vi "CRC16string气密机一.vi"(1 "数组":u16[](array[numeric]) format="%x") -> (0 "要发送的数据":string)   [LabVIEW 2014]
panel:
  out "交换后的校验和":u16 format="%x"
  out "校验和":i32 format="%x"
  out "数组个数":dbl
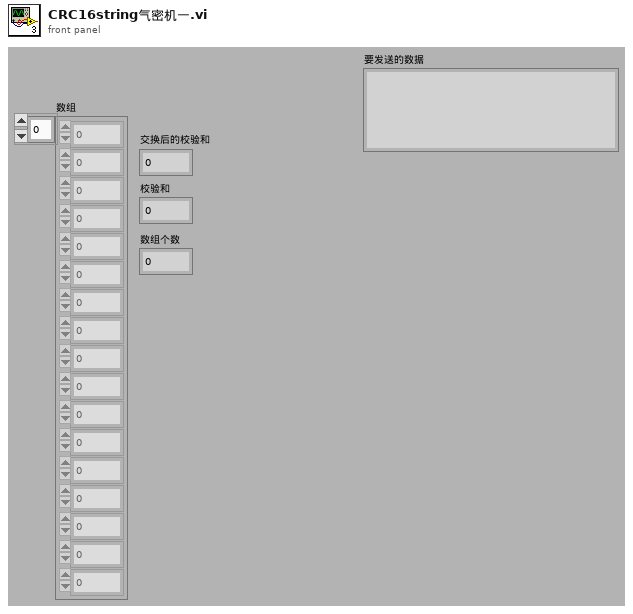
[diagram p1: front panel]
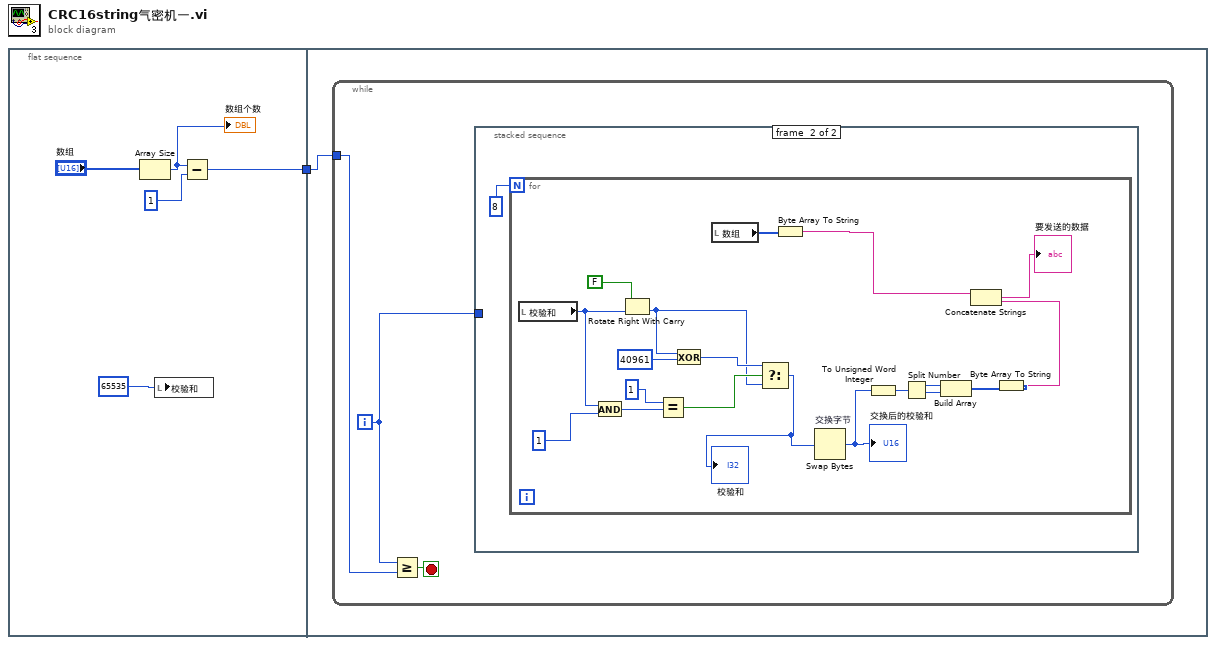
[diagram p0: block diagram]
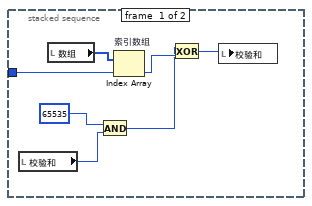
[diagram p2: hidden frame]
diagram:
  n1 = flat-sequence {
    tunnel: [w5] -> w1
    tunnel: w1 -> [w7]
    frame #0 {
      n2 = Array Size(array="数组") -> (size(s)=w2:i32)
      "数组个数" <- w2
      n3 = local write "校验和"(65535) -> ()
      n4 = Subtract(x=w2, y=1) -> (x-y=w5:i32)
    }
    frame #1 {
      n5 = while {
        tunnel: w7 -> [w9]
        i -> [w8]
        stop <- w10 stop-if-true
        n6 = Greater Or Equal?(x=w8, y=w9) -> (x >= y?=w10:bool)
        n7 = stacked-sequence {
          tunnel: w8 -> [w11 _]
          frame #0 {
            n8 = local read "校验和"() -> (w13:i32)
            n9 = local read "数组"() -> (w17:u16[])
            n10 = And(x=65535, y=w13) -> (x .and. y?=w12:i32)
            n11 = Index Array "索引数组"(array=w17, index=w11) -> (element=w16:u16)
            n12 = Exclusive Or(1:w16, 2:w12) -> (0:w15:i32)
            n13 = local write "校验和"(w15) -> ()
          }
          frame #1 {
            n14 = for {
              N: 8 ("y") -> [_]
              n15 = local read "校验和"() -> (w35:i32)
              n16 = And(x=w35, y=1) -> (x .and. y?=w33:i32)
              n17 = Rotate Right With Carry(2:w35, 3:FALSE ("传递")) -> (0:w29:i32)  [unwired: 1 out]
              n18 = Equal?(x=1, y=w33) -> (x = y?=w31:bool)
              n19 = Exclusive Or(1:40961, 2:w29) -> (0:w30:i32)
              n20 = local read "数组"() -> (w27:u16[])
              n21 = Select(t=w30, s=w31, f=w29) -> (s? t:f=w28:i32)
              "校验和" <- w28
              n22 = Byte Array To String(unsigned byte array=w27) -> (string=w26:string)
              n23 = Swap Bytes "交换字节"(anything=w28) -> (byte swapped=w24:i32)
              "交换后的校验和" <- w24
              n24 = To Unsigned Word Integer(number=w24) -> (unsigned 16bit integer=w23:u16)
              n25 = Split Number(x=w23) -> (hi(x)=w22:u8, lo(x)=w21:u8)
              n26 = Build Array(w22, w21) -> (w20:u8[])
              n27 = Byte Array To String(unsigned byte array=w20) -> (string=w19:string)
              n28 = Concatenate Strings(w26, w19) -> (→"要发送的数据":string)
            }
          }
        }
      }
    }
  }
